vi "Read Instrument Driver Type.vi"(8 "error in":errorcluster, 11 "Plugin_Driver in":refnum<class "Plugin_Driver.lvclass">) -> (0 "error out":errorcluster, 2 "Instrument Driver.lvclass":refnum<class "Instrument Driver.lvclass">, 3 "Plugin_Driver out":refnum<class "Plugin_Driver.lvclass">)   [LabVIEW 2020, in "Plugin.lvlib" / "Plugin_Driver.lvclass"]
doc: "Read Instrument Driver Type"
uses:
  Plugin_Driver.lvclass
  Drivers/Instrument Driver/Instrument Driver.lvclass
  Plugin_Driver.lvclass/Plugin_Driver.ctl
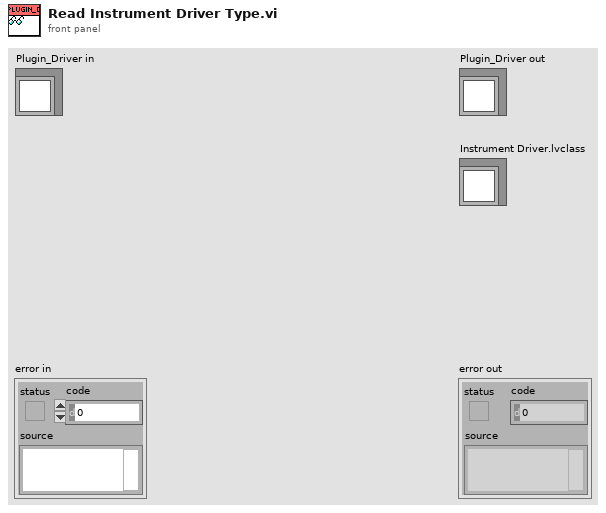
[diagram p1: front panel]
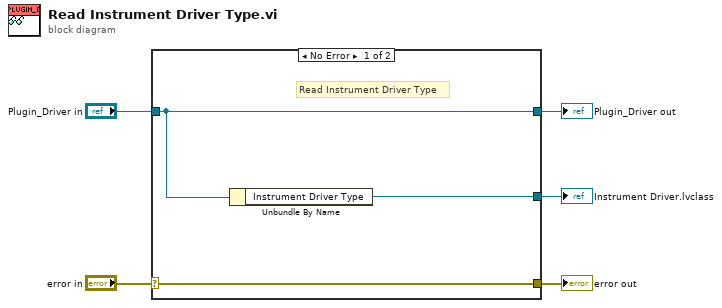
[diagram p0: block diagram]
diagram:
  n1 = case shown="No Error" "error in" {
    selector: "error in" -> [w8 w9]
    tunnel: [w8 w9] -> w4
    tunnel: [w7 w10] -> w2
    tunnel: "Plugin_Driver in" -> [w7 w10]
    tunnel: [w6 _] -> w1
    frame No Error {
      # "Read Instrument Driver Type"
      n2 = Unbundle By Name(w7) -> ("Instrument Driver Type"=w6:refnum<class "Instrument Driver.lvclass">)
    }
    frame Error {
    }
  }
  "error out" <- w4
  "Plugin_Driver out" <- w2
  "Instrument Driver.lvclass" <- w1
